vi "Plot Data.vi"(5 "Time Array":dbl[](array[numeric]), 7 "Device ID (0 index)":i32, 11 "Data Array":dbl[][](array[numeric])) -> (3 "Graph":cluster{"X":dbl, "Y":dbl}[](array[cluster]))   [LabVIEW 2017]
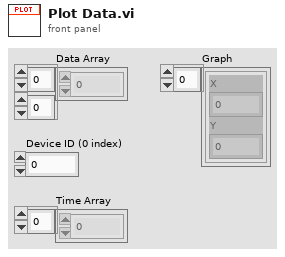
[diagram p1: front panel]
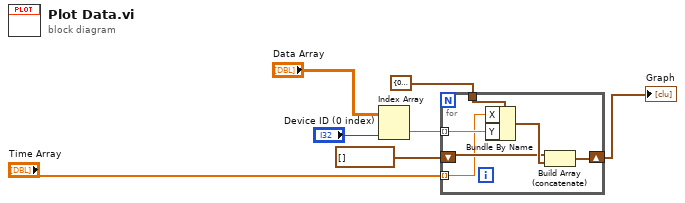
[diagram p0: block diagram]
diagram:
  n1 = Index Array(array="Data Array", index (col)="Device ID (0 index)") -> (element=w3:dbl[])  [unwired: 1 in]
  n2 = for {
    tunnel: w3 -> [w12] mode=indexing
    shift-right: [w9] -> w6
    shift-left: cluster{"X":dbl, "Y":dbl}[] [] ("Thermocouple 1") -> [w10]
    tunnel: cluster{"X":dbl, "Y":dbl} {"X"=0.0, "Y"=0.0} -> [w13]
    tunnel: "Time Array" -> [w8] mode=indexing
    n3 = Bundle By Name(cluster=w13, "X"=w8, "Y"=w12) -> (w11:cluster{"X":dbl, "Y":dbl})
    n4 = Build Array (concatenate)(w10, w11) -> (w9:cluster{"X":dbl, "Y":dbl}[])
  }
  "Graph" <- w6
